vi "SV Convert Complex Spectra to Data Object.vi"(0 "spectra":T7(array[cluster]) {"spectrum info"."x-axis units" items=["Time (s)"=0, "Frequency-CB (Hz)"=1, "Frequency-CPB (Hz)"=1248, "Frequency-Arbitrary (Hz)"=2357, "Quefrency (s)"=2, "Revolutions (rev)"=3, "Order"=4, "Speed (RPM)"=11, "Speed (rad/s)"=21, "Index"=65535]; "spectrum info"."weighting filter" items=["Linear", "A-weighting", "B-weighting", "C-weighting", "ITU-R 468-4", "Dolby", "CCITT", "C-message", "Wb", "Wc", "Wd", "We", "Wf", "Wh", "Wj", "Wk", "Wm", "AES17 20 kHz lowpass", "AES17 40 kHz lowpass", "AES17 20 kHz highpass", "AES17 40 kHz highpass"]; "spectrum info"."dB reference [EU]" format="%.2f"; "spectrum info"."engineering units" items=["custom..."=0, "V"=1, "A"=21, "C"=30, "pC"=31, "s"=32, "-"=29, "Pa"=2, "N"=20, "g"=3, "m/s^2"=4, "m/s"=5, "m"=6, "mm/s"=12, "mm"=13, "micron/s"=14, "micron"=15, "in/s^2"=7, "in/s"=8, "in"=9, "mil/s"=10, "mil"=11, "rad/s^2"=16, "rad/s"=17, "rad"=18, "deg/s^2"=26, "deg/s"=27, "deg"=28, "RPM"=22, "cycle/s^2"=23, "Hz"=24, "cycle"=25, "strain"=19]; "spectrum info"."spectral info"."window" items=["None "=0, "Hanning"=1, "Hamming"=2, "Blackman-Harris"=3, "Exact Blackman"=4, "Blackman"=5, "Flat Top"=6, "4 Term B-Harris "=7, "7 Term B-Harris"=8, "Low Sidelobe"=9, "Force - Exponential"=10, "Gaussian"=62]; "complex spectrum"."complex y" format="%.2f"; "complex spectrum"."df" format="%.2f"; "complex spectrum"."f0" format="%.2f"}, 5 "error in (no error)":errorcluster) -> (14 "Spectrum Data":refnum<class "Data.lvclass">, 19 "error out":errorcluster)   [LabVIEW 2017, in "Y (Complex) (N Ch).lvclass"]
doc: "Use this polymorphic VI to convert spectra to a class datatype that you can view on the Spectrum with Cursors XControl. You must manually select the polymorphic instance to use."
uses:
  <vilib>/addons/_NISVFA/_Shared subVIs/Data Objects/Y (Complex) (DBL)/Y (Complex) (N Ch).lvclass
  <vilib>/addons/_NISVFA/_Shared subVIs/Controls/svc_Spectrum Info.ctl
  <vilib>/addons/_NISVFA/_Shared subVIs/Controls/svc_X-Axis Units.ctl
  <vilib>/addons/_NISVFA/_Shared subVIs/Controls/svc_Spectrum Type.ctl
  <vilib>/addons/_NISVFA/_Shared subVIs/Controls/svc_Engineering Units Text Ring.ctl
  <vilib>/addons/_NISVFA/_Shared subVIs/Controls/svc_Weighting Filter Text Ring.ctl
  <vilib>/addons/_NISVFA/_Shared subVIs/Controls/svc_Complimentary Spectrum Units.ctl
  <vilib>/addons/_NISVFA/_Shared subVIs/Data Objects/Data/Data.lvclass
  C:/Program Files (x86)/National Instruments/LabVIEW 2017/vi.lib/addons/_NISVFA/_Shared subVIs/Data Objects/Data/Data.lvclass
  <vilib>/addons/_NISVFA/_Shared subVIs/Controls/NI Channel Properties.ctl
  <vilib>/addons/_NISVFA/_Shared subVIs/Data Objects/Y (Complex) (DBL)/Y (Complex) (N Ch).lvclass/Y (Complex) (N Ch).ctl
  <vilib>/addons/_NISVFA/_Shared subVIs/Data Objects/Data/Data.lvclass/Data.ctl
  <vilib>/addons/_NISVFA/_Shared subVIs/Data Objects/Data/Read Data Attributes.vi
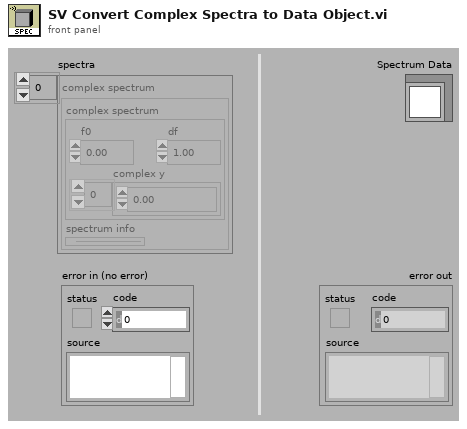
[diagram p1: front panel]
types:
  T1 = typedef "svc_Spectrum Info.ctl" = cluster{"channel name":string, "description":string, "x-axis units":T2, "spectral info":cluster{"spectrum type":T3, "linear/dB":enum16{"linear", "dB"}, "window":u16, "window size":i32, "FFT size":i32}, "engineering units":T4, "custom label":string, "dB reference [EU]":dbl, "peak units":enum16{"rms", "peak", "peak-peak"}, "weighting filter":T5, "spectral density?":bool, "unit label":string, "spectrum skewed?":bool, "complimentary spectrum units":T6}
  T2 = typedef "svc_X-Axis Units.ctl" = u16
  T3 = typedef "svc_Spectrum Type.ctl" = enum16{"FFT Spectrum [complex]", "Amplitude [Magnitude]", "Power [Magnitude^2]", "Cross Spectrum [complex]", "Frequency Response [Complex]"}
  T4 = typedef "svc_Engineering Units Text Ring.ctl" = u16
  T5 = typedef "svc_Weighting Filter Text Ring.ctl" = u16
  T6 = typedef "svc_Complimentary Spectrum Units.ctl" = enum16{"none", "radians", "degrees", "cycles", "imaginary"}
  T7 = cluster{"complex spectrum":cluster{"f0":dbl, "df":dbl, "complex y":cdb[]}, "spectrum info":T1}[]
  T8 = typedef "NI Channel Properties.ctl" = u16
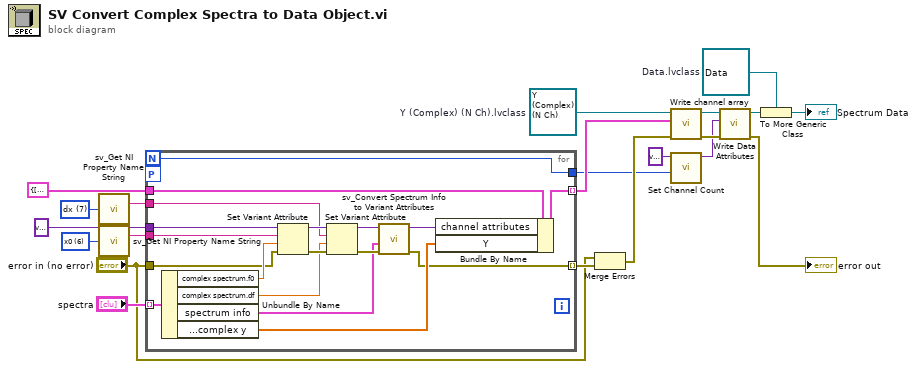
[diagram p0: block diagram]
diagram:
  w2 = T8 6 items=["Channel name", "Channel description", "Axis label", "Unit string", "Waveform X-axis label", "Waveform X-axis unit string", "x0", "dx", "Number of samples", "X channel", "Filter settled", "dB reference", "Window", "Window parameter", "Window size", "FFT size", "Peak units", "Spectrum type", "Magnitude scale", "Spectral density", "Sensor sensitivity (mV/EU)", "X-axis dimension", "LabVIEW datatype", "Function type", "Function subtype", "X values", "Independent channel", "Column index", "Collection name", "Collection ID", "X Columns", "Phase unwrapped"] ("property")
  w4 = T8 7 items=["Channel name", "Channel description", "Axis label", "Unit string", "Waveform X-axis label", "Waveform X-axis unit string", "x0", "dx", "Number of samples", "X channel", "Filter settled", "dB reference", "Window", "Window parameter", "Window size", "FFT size", "Peak units", "Spectrum type", "Magnitude scale", "Spectral density", "Sensor sensitivity (mV/EU)", "X-axis dimension", "LabVIEW datatype", "Function type", "Function subtype", "X values", "Independent channel", "Column index", "Collection name", "Collection ID", "X Columns", "Phase unwrapped"] ("property")
  w10 = refnum<class "Y (Complex) (N Ch).lvclass"> refnum  # Y (Complex) (N Ch).lvclass
  w20 = refnum<class "Data.lvclass"> refnum  # Data.lvclass
  n1 = call <vilib>:"sv_Get NI Property Name String.vi"("property"=w4) -> ("TDMS property name"=w3:string)  [unwired: 13 in, 1 out]
  n2 = call <vilib>:"sv_Get NI Property Name String.vi"("property"=w2) -> ("TDMS property name"=w1:string)  [unwired: 13 in, 1 out]
  n3 = for {
    N -> [w24]
    tunnel: "spectra" -> [w39] mode=indexing
    tunnel: variant ("data attributes") -> [w32]
    tunnel: cluster{"Y":cdb[], "channel attributes":variant} {"Y"=[], "channel attributes"=variant} ("channel data") -> [w31]
    tunnel: [w28] -> w16 mode=indexing
    workers-P: _ -> [_]
    tunnel: "error in (no error)" -> [w27]
    tunnel: [w26] -> w11 mode=indexing
    tunnel: [w24] -> w6
    tunnel: w3 -> [w23]
    tunnel: w1 -> [w22]
    n4 = Unbundle By Name(w39) -> ("complex spectrum.f0"=w34:dbl, "complex spectrum.df"=w33:dbl, "spectrum info"=w25:T1, "complex spectrum.complex y"=w29:cdb[])
    n5 = Set Variant Attribute(Variant=w32, name=w22, value=w34, error in=w27) -> (Variant out=w36:variant, error out=w37:errorcluster)  [unwired: 1 out]
    n6 = Set Variant Attribute(Variant=w36, name=w23, value=w33, error in=w37) -> (Variant out=w38:variant, error out=w35:errorcluster)  [unwired: 1 out]
    n7 = call <vilib>:"sv_Convert Spectrum Info to Variant Attributes.vi"("error in"=w35, "spectrum info"=w25, "attributes in"=w38) -> ("error out"=w26:errorcluster, "attributes out"=w30:variant)  [unwired: 5 in, 2 out]
    n8 = Bundle By Name(cluster=w31, "channel attributes"=w30, "Y"=w29) -> (w28:cluster{"Y":cdb[], "channel attributes":variant})
  }
  n9 = Merge Errors("error in (no error)", w11) -> (w9:errorcluster)
  n10 = call <vilib>:"Write channel array.vi"("error in (no error)"=w9, "channel array"=w16, "Y (Complex) (N Ch) in"=w10) -> ("error out"=w14:errorcluster, "Y (Complex) (N Ch) out"=w15:refnum<class "Y (Complex) (N Ch).lvclass">)  [unwired: 7 in]
  n11 = call <vilib>:"Set Channel Count.vi"("number of channels"=w6, "variant in"=variant ("data attributes")) -> ("variant out"=w7:variant)  [unwired: 9 in]
  n12 = call <vilib>:"Write Data Attributes.vi"("error in (no error)"=w14, "data attributes"=w7, "Data in"=w15) -> ("error out"=→"error out":errorcluster, "Data out"=w13:refnum<class "Y (Complex) (N Ch).lvclass">)  [unwired: 7 in]
  n13 = To More Generic Class(target class=w20, reference=w13) -> (generic class reference=→"Spectrum Data":refnum<class "Data.lvclass">)
